vi "AlliGator Create Source Image ROI Grid.vi"(8 "Error In":errorcluster, 11 "ROI":T1 {"Contours"."Type" items=["No Selection", "Point", "Line", "Rectangle", "Oval", "Polygon", "Freehand Region", "Annulus", "Unused2", "Unused3", "Broken Line", "Freehand Line", "Rotated Rectangle"]}) -> (0 "Error Out":errorcluster, 2 "Message":string)   [LabVIEW 2021, in "AlliGator ROIs.lvlib"]
doc: "Creates a series of Source Image ROIs layed out on a grid."
uses:
  AlliGator ROIs.lvlib
  Image/ROI Bounds.ctl
  AlliGator ROI Manager Actions.ctl
  AlliGator Source Image ROI Storage [MULT] v3.vi
  Strings/Strings.lvlib
  Image/Image.lvlib
panel:
  # "see the AlliGator License on the block diagram (Ctrl+E or Window:Show Block Diagram)"
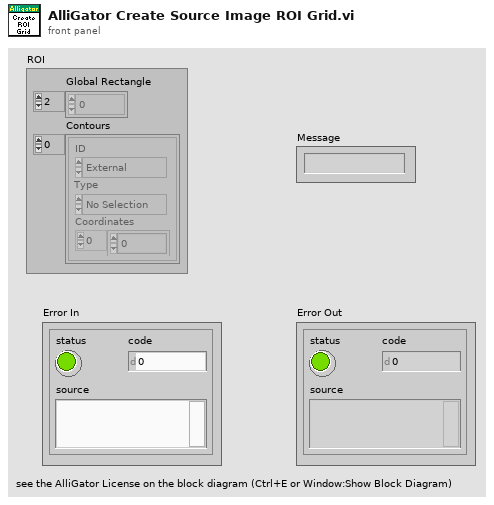
[diagram p1: front panel]
types:
  T1 = typedef "ROI Descriptor" = cluster{"Global Rectangle":i32[], "Contours":cluster{"ID":enum32{"External", "Internal"}, "Type":u32, "Coordinates":i32[]}[]}
  T2 = typedef "Image.lvlib/ROI Bounds.ctl" = cluster{"Ymax":i32, "Xmin":i32, "Ymin":i32, "Xmax":i32}
  T3 = typedef "Image.lvlib/ROI Grid Definition.ctl" = cluster{"Horizontal Step":i32, "Vertical Step":i32, "Horizontal Size":i32, "Vertical Size":i32, "# Horizontal ROIs":i32, "# Vertical ROIs":i32, "Definition by":bool, "ROI Type":T4}
  T4 = typedef "Image.lvlib/ROI  Type.ctl" = enum16{"Point", "Oval", "Rectangle"}
  T5 = typedef "AlliGator ROIs.lvlib/AlliGator ROI Manager Actions.ctl" = enum16{"Undefined", "Delete Current ROI", "Delete All Unselected ROIs", "Delete Multiple ROIs", "Delete All ROIs", "Swap ROIs", "Insert ROI", "Update Current ROI Descriptor", "Rename Current ROI", "Store New ROI", "Store Multiple ROIs", "Select Next ROI", "Select Previous ROI", "Find Selected ROI", "Show All ROIs", "Update ROI Manager Window", "Merge All ROIs", "Unmerge ROI", "Set Selected ROI by ID"}
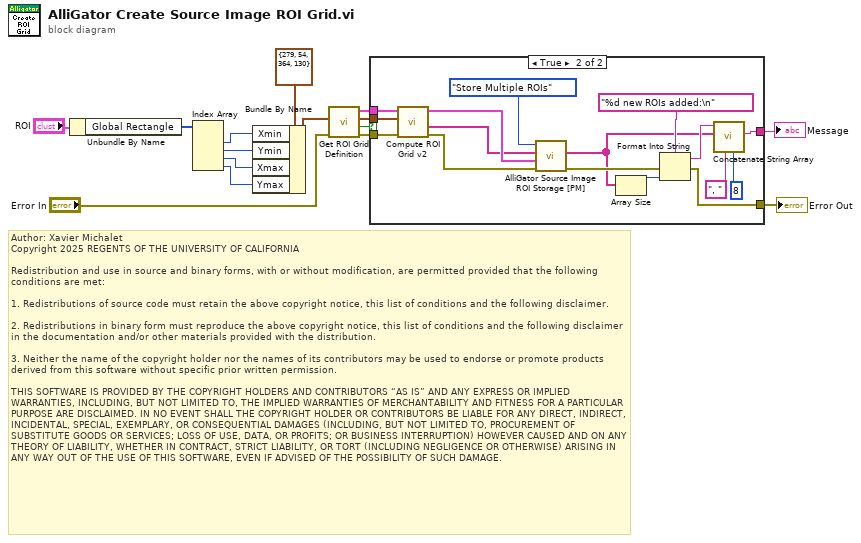
[diagram p0: block diagram]
diagram:
  # "Author: Xavier Michalet\nCopyright 2025 REGENTS OF THE UNIVERSITY OF CALIFORNIA\n\nRedistribution and use in source and binary forms, with or without modification, are permitted provided that the following conditions are met:\n\n1. Redistributions of source code must retain the above copyright notice, this list of conditions and the following disclaimer.\n\n2. Redistributions in binary form must reproduce the above copyright notice, this list of conditions and the following disclaimer in the documentation and/or other materials provided with the distribution.\n\n3. Neither the name of the copyright holder nor the names of its contributors may be used to endorse or promote products derived from this software without specific prior written permission.\n\nTHIS SOFTWARE IS PROVIDED BY THE COPYRIGHT HOLDERS AND CONTRIBUTORS “AS IS” AND ANY EXPRESS OR IMPLIED WARRANTIES, INCLUDING, BUT NOT LIMITED TO, THE IMPLIED WARRANTIES OF MERCHANTABILITY AND FITNESS FOR A PARTICULAR PURPOSE ARE DISCLAIMED. IN NO EVENT SHALL THE COPYRIGHT HOLDER OR CONTRIBUTORS BE LIABLE FOR ANY DIRECT, INDIRECT, INCIDENTAL, SPECIAL, EXEMPLARY, OR CONSEQUENTIAL DAMAGES (INCLUDING, BUT NOT LIMITED TO, PROCUREMENT OF SUBSTITUTE GOODS OR SERVICES; LOSS OF USE, DATA, OR PROFITS; OR BUSINESS INTERRUPTION) HOWEVER CAUSED AND ON ANY THEORY OF LIABILITY, WHETHER IN CONTRACT, STRICT LIABILITY, OR TORT (INCLUDING NEGLIGENCE OR OTHERWISE) ARISING IN ANY WAY OUT OF THE USE OF THIS SOFTWARE, EVEN IF ADVISED OF THE POSSIBILITY OF SUCH DAMAGE."
  n1 = Unbundle By Name("ROI") -> ("Global Rectangle"=w7:i32[])
  n2 = Index Array(array=w7) -> (element #1=w6:i32, element #2=w5:i32, element #3=w4:i32, element #4=w3:i32)  [unwired: 4 in]
  n3 = Bundle By Name(cluster=T2 {"Ymax"=279, "Xmin"=54, "Ymin"=364, "Xmax"=130} ("Current ROI Bounds"), "Xmin"=w6, "Ymin"=w5, "Xmax"=w4, "Ymax"=w3) -> (w8:T2)
  n4 = call "Get ROI Grid Definition.vi"("error in (no error)"="Error In", "Current ROI Bounds"=w8) -> ("error out"=w10:errorcluster, "OK"=w13:bool, "ROI Bounds out"=w11:T2, "Grid Definition"=w12:T3)  [unwired: 6 in]
  n5 = case shown="True" w13 {
    tunnel: [w16 w19] -> w2
    tunnel: [_ w32] -> w1
    tunnel: w12 -> [_ w28]
    tunnel: w11 -> [_ w26]
    tunnel: w10 -> [w16 w25]
    frame False {
    }
    frame True {
      n6 = call "Compute ROI Grid v2.vi"("Error In"=w25, "Current ROI Bounds"=w26, "Grid Definition"=w28) -> ("Error Out"=w24:errorcluster, "ROI Names"=w23:string[], "Current ROI Descriptor"=w27:T1[])  [unwired: 6 in]
      n7 = call-poly "AlliGator Source Image ROI Storage [PM].vi"("Error In"=w24, "Current ROI Descriptors"=w27, "Default Names (\"ROI\")"=w23, "Action"=AlliGator_ROI_Manager_Actions."Store Multiple ROIs") -> ("Error Out"=w20:errorcluster, "Current ROI Names"=w18:string[])  [unwired: 2 in, 4 out]
      n8 = Array Size(array=w18) -> (size(s)=w30:i32)
      n9 = Format Into String(format string="%d new ROIs added:\n" ("Prefix (\"\")"), error in=w20, w30) -> (resulting string=w31:string, error out=w19:errorcluster)  [unwired: 1 in]
      n10 = call "Concatenate String Array.vi"("Max Number of Elements (None: -1)"=8 ("Max Number of Elements (None: 1)"), "Separator (TAB)"=", ", "String Array"=w18, "Prefix (\"\")"=w31) -> ("Formatted String"=w32:string)  [unwired: 7 in]
    }
  }
  "Error Out" <- w2
  "Message" <- w1
